vi "REPLACE.vi"(7 "Actor in":refnum<class "Actor.lvclass">, 11 "Msg State in":refnum<class "Msg State.lvclass">) -> (2 "Destroy?":bool, 5 "Actor out":refnum<class "Actor.lvclass">)   [LabVIEW 2021, in "jettl.lvlib" / "Msg State.lvclass"]
uses:
  Msg State.lvclass
  Actor/Actor/Actor.lvclass
  Actor/Msgs/Destroy/Destroy Msg/Destroy Msg.lvclass
  C:/git/jettl/src/Actor/Msg/Msg.lvclass
  Msg State.lvclass/Msg State.ctl
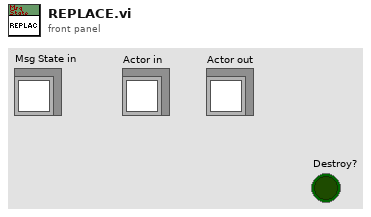
[diagram p1: front panel]
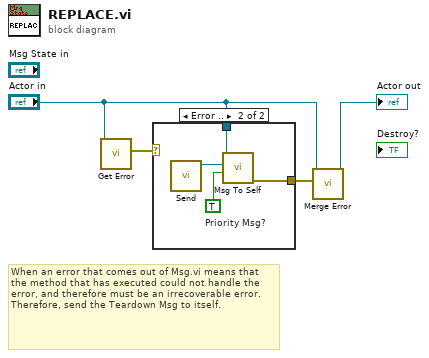
[diagram p0: block diagram]
diagram:
  # "When an error that comes out of Msg.vi means that the method that has executed could not handle the error, and therefore must be an irrecoverable error. Therefore, send the Teardown Msg to itself."
  n1 = call-dynamic "Get Error.vi"("Actor in"="Actor in") -> ("Error"=w4:errorcluster)  [unwired: 10 in]
  n2 = case shown="Error .." w4 {
    tunnel: "Actor in" -> [_ w8]
    tunnel: [_ w5] -> w3
    frame No Error {
    }
    frame Error {
      w6 = TRUE  # Priority Msg?
      n3 = call "Send.vi"() -> ("Destroy Msg out"=w7:refnum<class "Destroy Msg.lvclass">)  [unwired: 11 in]
      n4 = call-dynamic "Msg To Self.vi"("Priority Msg?"=w6, "Msg"=w7, "Actor in"=w8) -> ("error out"=w5:errorcluster)  [unwired: 8 in]
    }
  }
  n5 = call-dynamic "Merge Error.vi"("Error"=w3, "Set Error in"="Actor in") -> ("Set Error out"=→"Actor out":refnum<class "Actor.lvclass">)  [unwired: 9 in]
